vi "error.Read code.vi"(8 "error in (no error)":errorcluster, 11 "error in":refnum<class "error.lvclass">) -> (0 "error out":errorcluster, 2 "code":i32, 3 "error out":refnum<class "error.lvclass">)   [LabVIEW 2016, in "error.lvclass"]
uses:
  error.lvclass
  error.lvclass/error.ctl
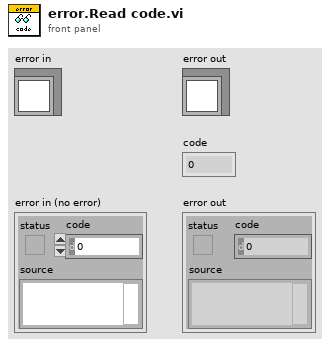
[diagram p1: front panel]
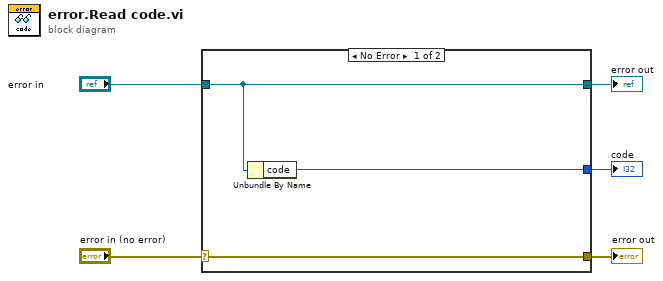
[diagram p0: block diagram]
diagram:
  n1 = case shown="No Error" "error in (no error)" {
    selector: "error in (no error)" -> [w8 w9]
    tunnel: [w8 w9] -> w4
    tunnel: [w7 w10] -> w2
    tunnel: "error in" -> [w7 w10]
    tunnel: [w6 _] -> w1
    frame No Error {
      n2 = Unbundle By Name(w7) -> ("code"=w6:i32)
    }
    frame Error {
    }
  }
  "error out" <- w4
  "error out" <- w2
  "code" <- w1
